vi "Autonomous Independent.vi"() -> ()   [LabVIEW 2016]
doc: "This VI is called when autonomous begins, and will automatically be terminated when autonomous ends. You can carry out timed or sensor driven robot movement independently without needing to return to the caller."
uses:
  <vilib>/Rock Robotics/WPI/ThirdParty/CanMotor/TalonSRX/WPI_CANTalonSRX_GlobalStatus.ctl
  <vilib>/Rock Robotics/WPI/SafetyOutput/WPI_SafetyOutputConfigMenu.ctl
panel:
  in  "y":dbl
  in  "Distance 2":dbl=6.462
  in  "Effort 2":dbl=0.5 format="%#_13g"
  out "Talon SRX Status 2":T1
  out "Talon SRX Status":T1
  in  "Effort 1":dbl=0.5 format="%#_13g"
  in  "Distance 1":dbl=6.462
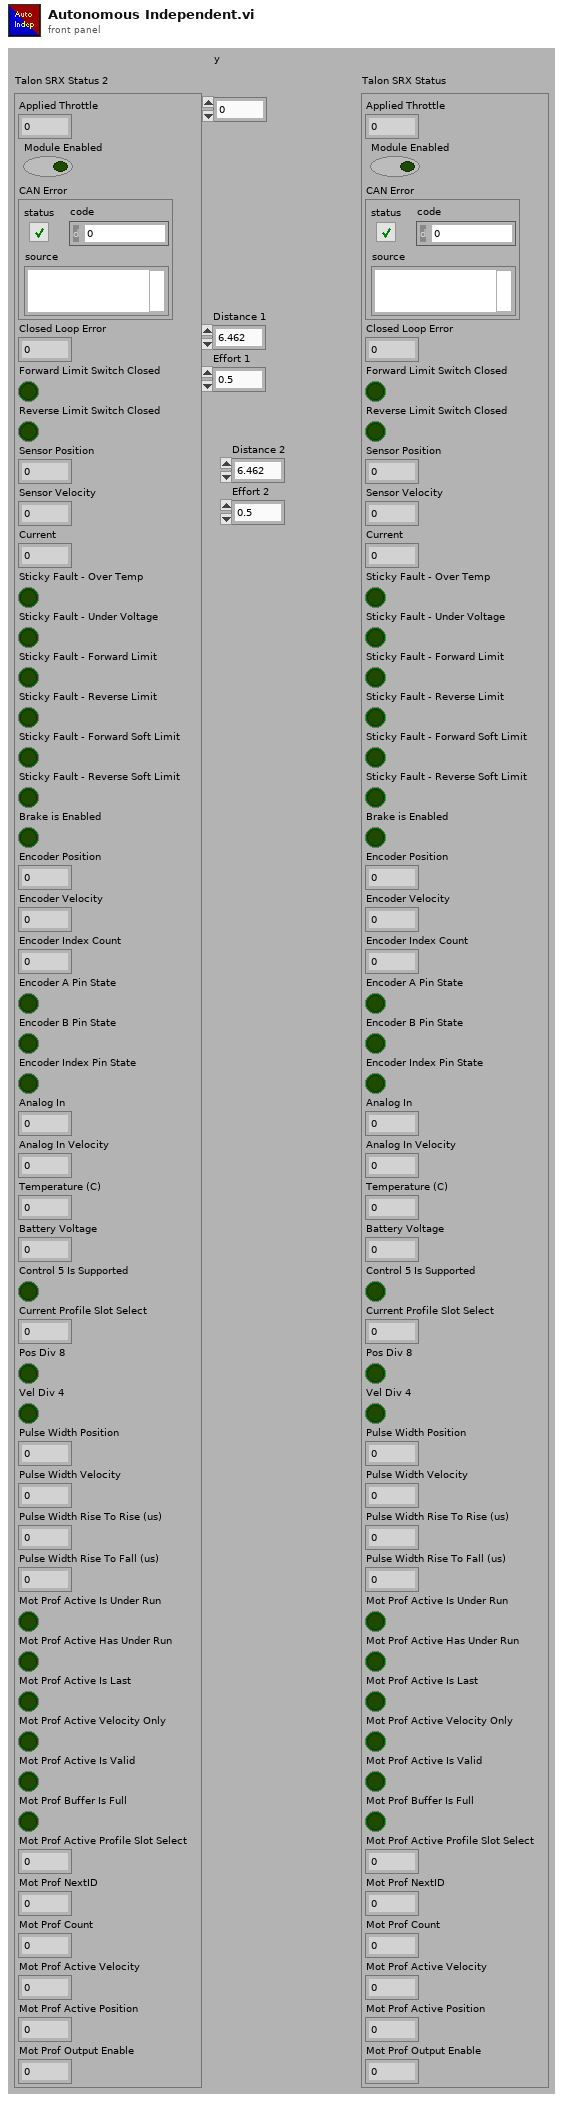
[diagram p1: front panel]
types:
  T1 = typedef "WPI_CANTalonSRX_GlobalStatus.ctl" = cluster{"Applied Throttle":dbl, "Module Enabled":bool, "CAN Error":errorcluster, "Closed Loop Error":dbl, "Forward Limit Switch Closed":bool, "Reverse Limit Switch Closed":bool, "Sensor Position":dbl, "Sensor Velocity":dbl, "Current":dbl, "Sticky Fault - Over Temp":bool, "Sticky Fault - Under Voltage":bool, "Sticky Fault - Forward Limit":bool, "Sticky Fault - Reverse Limit":bool, "Sticky Fault - Forward Soft Limit":bool, "Sticky Fault - Reverse Soft Limit":bool, "Brake is Enabled":bool, "Encoder Position":dbl, "Encoder Velocity":dbl, "Encoder Index Count":dbl, "Encoder A Pin State":bool, "Encoder B Pin State":bool, "Encoder Index Pin State":bool, "Analog In":dbl, "Analog In Velocity":dbl, "Temperature (C)":dbl, "Battery Voltage":dbl, "Control 5 Is Supported":bool, "Current Profile Slot Select":dbl, "Pos Div 8":bool, "Vel Div 4":bool, "Pulse Width Position":i32, "Pulse Width Velocity":i32, "Pulse Width Rise To Rise (us)":i32, "Pulse Width Rise To Fall (us)":i32, "Mot Prof Active Is Under Run":bool, "Mot Prof Active Has Under Run":bool, "Mot Prof Active Is Last":bool, "Mot Prof Active Velocity Only":bool, "Mot Prof Active Is Valid":bool, "Mot Prof Buffer Is Full":bool, "Mot Prof Active Profile Slot Select":i32, "Mot Prof NextID":i32, "Mot Prof Count":i32, "Mot Prof Active Velocity":dbl, "Mot Prof Active Position":dbl, "Mot Prof Output Enable":i32}
  T2 = typedef "WPI_SafetyOutputConfigMenu.ctl" = enum16{"Enable", "Disable"}
  T3 = typedef "WPI_MotorControlDeviceRef.ctl" = cluster{"DeviceStatus":errorcluster, "Type":T4, "PWM":cluster{"PWM Channel":T5, "DeadBand":T6}, "CAN":cluster{"Device Number":u8, "SetOutput VI Ref":variant, "GetOutput VI Ref":variant, "Enable VI Ref":variant, "Disable VI Ref":variant, "Data":variant}, "Invert":bool}
  T4 = typedef "WPI_MotorControlType.ctl" = enum16{"PWM", "CAN"}
  T5 = typedef "FPGA_DIOPWMChannel.ctl" = enum8{"PWM 0", "PWM 1", "PWM 2", "PWM 3", "PWM 4", "PWM 5", "PWM 6", "PWM 7", "PWM 8", "PWM 9", "PWM MXP 0", "PWM MXP 1", "PWM MXP 2", "PWM MXP 3", "PWM MXP 4", "PWM MXP 5", "PWM MXP 6", "PWM MXP 7", "PWM MXP 8", "PWM MXP 9", "Invalid"}
  T6 = typedef "WPI_PWMDeadband.ctl" = cluster{"Name":string, "maxPositivePwm":i32, "minPositivePwm":i32, "centerPwm":i32, "maxNegativePwm":i32, "minNegativePwm":i32, "angularRange":u16}
  T7 = typedef "WPI_GyroDevRef.ctl" = cluster{"DevStatus":errorcluster, "Analog Channel":T8, "Offset":dbl, "Gain (VoltsPerDegree/Second)":dbl, "Gyro Type":enum16{"Analog", "XRS450"}, "Handle":i32, "SPI Bus":T9, "Device Found":bool, "Sample Rate":dbl, "Calibrate On Open":bool}
  T8 = typedef "FPGA_AIChannel.ctl" = enum8{"AI 0", "AI 1", "AI 2", "AI 3", "AI MXP 0", "AI MXP 1", "AI MXP 2", "AI MXP 3", "Invalid"}
  T9 = typedef "spi_bus.ctl" = enum16{"SPI On-Board, CS0", "SPI On-Board, CS1", "SPI On-Board, CS2", "SPI On-Board, CS3", "SPI MXP", "Invalid"}
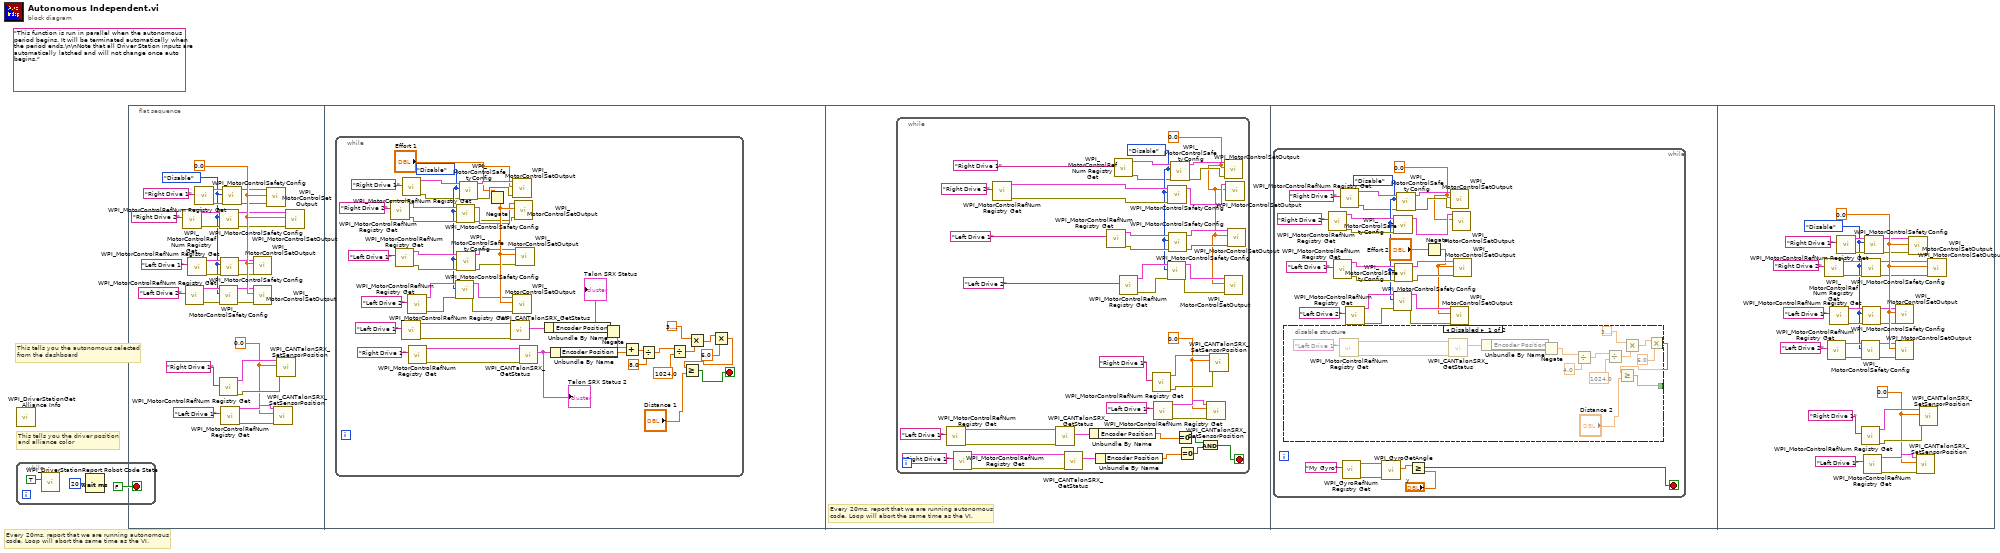
[diagram p0: block diagram]
diagram:
  (unwired) "This function is run in parallel when the autonomous period begins. It will be terminated automatically when the period ends.\n\nNote that all Driver Station inputs are automatically latched and will not change once auto begins."
  # "This tells you the autonomous selected\nfrom the dashboard"
  # "Every 20ms, report that we are running autonomous\ncode. Loop will abort the same time as the VI."
  # "This tells you the driver position\nand alliance color"
  n1 = while {
    stop <- FALSE stop-if-true
    n2 = call <vilib>:"WPI_DriverStationReport Robot Code State.vi"("Autonomous"=TRUE) -> ()  [unwired: 10 in, 1 out]
    n3 = Wait (ms)(milliseconds to wait=u32 20) -> ()  [unwired: 1 out]
  }
  n4 = call <vilib>:"WPI_DriverStationGet Alliance Info.vi"() -> ()  [unwired: 12 out]
  n5 = flat-sequence {
    frame #0 {
      w12 = WPI_SafetyOutputConfigMenu."Disable" ("mode")
      w21 = 0.0 ("Effort 2")
      w26 = 0.0 ("New Sensor Position")
      n6 = call <vilib>:"WPI_MotorControlRefNum Registry Get.vi"("refnum name"="Right Drive 2") -> ("error out"=w17:errorcluster, "MotorControlDevRef"=w18:T3)  [unwired: 9 in]
      n7 = call <vilib>:"WPI_MotorControlRefNum Registry Get.vi"("refnum name"="Left Drive 2") -> ("error out"=w13:errorcluster, "MotorControlDevRef"=w14:T3)  [unwired: 9 in]
      n8 = call <vilib>:"WPI_MotorControlRefNum Registry Get.vi"("refnum name"="Left Drive 1") -> ("error out"=w15:errorcluster, "MotorControlDevRef"=w16:T3)  [unwired: 9 in]
      n9 = call <vilib>:"WPI_MotorControlRefNum Registry Get.vi"("refnum name"="Right Drive 1") -> ("error out"=w20:errorcluster, "MotorControlDevRef"=w19:T3)  [unwired: 9 in]
      n10 = call <vilib>:"WPI_MotorControlSafetyConfig.vi"("error in (no error)"=w13, "mode"=w12, "MotorControlDevRef"=w14) -> ("error out"=w4:errorcluster, "MotorControlDevRef"=w5:T3)  [unwired: 7 in]
      n11 = call <vilib>:"WPI_MotorControlRefNum Registry Get.vi"("refnum name"="Right Drive 1") -> ("error out"=w27:errorcluster, "MotorControlDevRef"=w28:T3)  [unwired: 9 in]
      n12 = call <vilib>:"WPI_MotorControlSafetyConfig.vi"("error in (no error)"=w17, "mode"=w12, "MotorControlDevRef"=w18) -> ("error out"=w8:errorcluster, "MotorControlDevRef"=w9:T3)  [unwired: 7 in]
      n13 = call <vilib>:"WPI_MotorControlSafetyConfig.vi"("error in (no error)"=w15, "mode"=w12, "MotorControlDevRef"=w16) -> ("error out"=w6:errorcluster, "MotorControlDevRef"=w7:T3)  [unwired: 7 in]
      n14 = call <vilib>:"WPI_MotorControlRefNum Registry Get.vi"("refnum name"="Left Drive 1") -> ("error out"=w29:errorcluster, "MotorControlDevRef"=w30:T3)  [unwired: 9 in]
      n15 = call <vilib>:"WPI_MotorControlSafetyConfig.vi"("error in (no error)"=w20, "mode"=w12, "MotorControlDevRef"=w19) -> ("error out"=w10:errorcluster, "MotorControlDevRef"=w11:T3)  [unwired: 7 in]
      n16 = call <vilib>:"WPI_MotorControlSetOutput.vi"("error in (no error)"=w6, "Output"=w21, "MotorControlDevRef"=w7) -> ()  [unwired: 6 in, 3 out]
      n17 = call <vilib>:"WPI_MotorControlSetOutput.vi"("error in (no error)"=w4, "Output"=w21, "MotorControlDevRef"=w5) -> ()  [unwired: 6 in, 3 out]
      n18 = call <vilib>:"WPI_MotorControlSetOutput.vi"("error in (no error)"=w10, "Output"=w21, "MotorControlDevRef"=w11) -> ()  [unwired: 6 in, 3 out]
      n19 = call <vilib>:"WPI_CANTalonSRX_SetSensorPosition.vi"("error in (no error)"=w29, "New Sensor Position"=w26, "CAN Talon SRX Ref"=w30) -> ()  [unwired: 7 in, 2 out]
      n20 = call <vilib>:"WPI_CANTalonSRX_SetSensorPosition.vi"("error in (no error)"=w27, "New Sensor Position"=w26, "CAN Talon SRX Ref"=w28) -> ()  [unwired: 7 in, 2 out]
      n21 = call <vilib>:"WPI_MotorControlSetOutput.vi"("error in (no error)"=w8, "Output"=w21, "MotorControlDevRef"=w9) -> ()  [unwired: 6 in, 3 out]
    }
    frame #1 {
      n22 = while {
        stop <- w42 stop-if-true
        w48 = WPI_SafetyOutputConfigMenu."Disable" ("mode")
        n23 = call <vilib>:"WPI_MotorControlRefNum Registry Get.vi"("refnum name"="Right Drive 2") -> ("error out"=w51:errorcluster, "MotorControlDevRef"=w52:T3)  [unwired: 9 in]
        n24 = call <vilib>:"WPI_MotorControlRefNum Registry Get.vi"("refnum name"="Left Drive 1") -> ("error out"=w55:errorcluster, "MotorControlDevRef"=w56:T3)  [unwired: 9 in]
        n25 = call <vilib>:"WPI_MotorControlRefNum Registry Get.vi"("refnum name"="Left Drive 1") -> ("error out"=w76:errorcluster, "MotorControlDevRef"=w77:T3)  [unwired: 9 in]
        n26 = call <vilib>:"WPI_MotorControlRefNum Registry Get.vi"("refnum name"="Right Drive 1") -> ("error out"=w46:errorcluster, "MotorControlDevRef"=w63:T3)  [unwired: 9 in]
        n27 = call <vilib>:"WPI_MotorControlRefNum Registry Get.vi"("refnum name"="Left Drive 2") -> ("error out"=w59:errorcluster, "MotorControlDevRef"=w60:T3)  [unwired: 9 in]
        n28 = call <vilib>:"WPI_MotorControlRefNum Registry Get.vi"("refnum name"="Right Drive 1") -> ("error out"=w40:errorcluster, "MotorControlDevRef"=w74:T3)  [unwired: 9 in]
        n29 = call <vilib>:"WPI_MotorControlSafetyConfig.vi"("error in (no error)"=w59, "mode"=w48, "MotorControlDevRef"=w60) -> ("error out"=w57:errorcluster, "MotorControlDevRef"=w58:T3)  [unwired: 7 in]
        n30 = call <vilib>:"WPI_MotorControlSafetyConfig.vi"("error in (no error)"=w51, "mode"=w48, "MotorControlDevRef"=w52) -> ("error out"=w49:errorcluster, "MotorControlDevRef"=w50:T3)  [unwired: 7 in]
        n31 = call <vilib>:"WPI_MotorControlSafetyConfig.vi"("error in (no error)"=w55, "mode"=w48, "MotorControlDevRef"=w56) -> ("error out"=w53:errorcluster, "MotorControlDevRef"=w54:T3)  [unwired: 7 in]
        n32 = call <vilib>:"WPI_MotorControlSafetyConfig.vi"("error in (no error)"=w46, "mode"=w48, "MotorControlDevRef"=w63) -> ("error out"=w47:errorcluster, "MotorControlDevRef"=w62:T3)  [unwired: 7 in]
        n33 = Negate(x="Effort 1") -> (-x=w61:dbl)
        n34 = call <vilib>:"WPI_CANTalonSRX_GetStatus.vi"("error in (no error)"=w76, "CAN Talon SRX Ref"=w77) -> ("Talon SRX Status"=w75:T1)  [unwired: 7 in, 2 out]
        "Talon SRX Status" <- w75
        n35 = call <vilib>:"WPI_MotorControlSetOutput.vi"("error in (no error)"=w47, "Output"="Effort 1", "MotorControlDevRef"=w62) -> ()  [unwired: 6 in, 3 out]
        n36 = call <vilib>:"WPI_MotorControlSetOutput.vi"("error in (no error)"=w57, "Output"=w61, "MotorControlDevRef"=w58) -> ()  [unwired: 6 in, 3 out]
        n37 = call <vilib>:"WPI_MotorControlSetOutput.vi"("error in (no error)"=w49, "Output"=w61, "MotorControlDevRef"=w50) -> ()  [unwired: 6 in, 3 out]
        n38 = call <vilib>:"WPI_MotorControlSetOutput.vi"("error in (no error)"=w53, "Output"=w61, "MotorControlDevRef"=w54) -> ()  [unwired: 6 in, 3 out]
        n39 = call <vilib>:"WPI_CANTalonSRX_GetStatus.vi"("error in (no error)"=w40, "CAN Talon SRX Ref"=w74) -> ("Talon SRX Status"=w44:T1)  [unwired: 7 in, 2 out]
        "Talon SRX Status 2" <- w44
        n40 = Unbundle By Name(w75) -> ("Encoder Position"=w66:dbl)
        n41 = Unbundle By Name(w44) -> ("Encoder Position"=w67:dbl)
        n42 = Negate(x=w66) -> (-x=w43:dbl)
        n43 = Add(x=w43, y=w67) -> (x+y=w65:dbl)
        n44 = Divide(x=w65, y=8.0) -> (x/y=w39:dbl)
        n45 = Divide(x=w39, y=1024.0) -> (x/y=w36:dbl)
        n46 = Multiply(x=3.141592653589793, y=w36) -> (x*y=w37:dbl)
        n47 = Multiply(x=w37, y=6.0) -> (x*y=w33:dbl)
        n48 = Greater Or Equal?(x=w33, y="Distance 1") -> (x >= y?=w42:bool)
      }
    }
    frame #2 {
      # "Every 20ms, report that we are running autonomous\ncode. Loop will abort the same time as the VI."
      n49 = while {
        stop <- w78 stop-if-true
        w91 = 0.0
        w95 = WPI_SafetyOutputConfigMenu."Disable" ("mode")
        w112 = 0.0 ("New Sensor Position")
        n50 = call <vilib>:"WPI_MotorControlRefNum Registry Get.vi"("refnum name"="Left Drive 1") -> ("error out"=w89:errorcluster, "MotorControlDevRef"=w90:T3)  [unwired: 9 in]
        n51 = call <vilib>:"WPI_MotorControlRefNum Registry Get.vi"("refnum name"="Right Drive 1") -> ("error out"=w83:errorcluster, "MotorControlDevRef"=w87:T3)  [unwired: 9 in]
        n52 = call <vilib>:"WPI_MotorControlRefNum Registry Get.vi"("refnum name"="Right Drive 2") -> ("error out"=w96:errorcluster, "MotorControlDevRef"=w97:T3)  [unwired: 9 in]
        n53 = call <vilib>:"WPI_CANTalonSRX_GetStatus.vi"("error in (no error)"=w89, "CAN Talon SRX Ref"=w90) -> ("Talon SRX Status"=w88:T1)  [unwired: 7 in, 2 out]
        n54 = call <vilib>:"WPI_CANTalonSRX_GetStatus.vi"("error in (no error)"=w83, "CAN Talon SRX Ref"=w87) -> ("Talon SRX Status"=w84:T1)  [unwired: 7 in, 2 out]
        n55 = Unbundle By Name(w88) -> ("Encoder Position"=w82:dbl)
        n56 = Unbundle By Name(w84) -> ("Encoder Position"=w80:dbl)
        n57 = call <vilib>:"WPI_MotorControlRefNum Registry Get.vi"("refnum name"="Left Drive 1") -> ("error out"=w100:errorcluster, "MotorControlDevRef"=w101:T3)  [unwired: 9 in]
        n58 = call <vilib>:"WPI_MotorControlRefNum Registry Get.vi"("refnum name"="Right Drive 1") -> ("error out"=w93:errorcluster, "MotorControlDevRef"=w107:T3)  [unwired: 9 in]
        n59 = call <vilib>:"WPI_MotorControlRefNum Registry Get.vi"("refnum name"="Left Drive 2") -> ("error out"=w104:errorcluster, "MotorControlDevRef"=w105:T3)  [unwired: 9 in]
        n60 = call <vilib>:"WPI_MotorControlRefNum Registry Get.vi"("refnum name"="Right Drive 1") -> ("error out"=w113:errorcluster, "MotorControlDevRef"=w114:T3)  [unwired: 9 in]
        n61 = call <vilib>:"WPI_MotorControlRefNum Registry Get.vi"("refnum name"="Left Drive 1") -> ("error out"=w115:errorcluster, "MotorControlDevRef"=w116:T3)  [unwired: 9 in]
        n62 = call <vilib>:"WPI_MotorControlSafetyConfig.vi"("error in (no error)"=w104, "mode"=w95, "MotorControlDevRef"=w105) -> ("error out"=w102:errorcluster, "MotorControlDevRef"=w103:T3)  [unwired: 7 in]
        n63 = call <vilib>:"WPI_MotorControlSafetyConfig.vi"("error in (no error)"=w96, "mode"=w95, "MotorControlDevRef"=w97) -> ("MotorControlDevRef"=w92:T3)  [unwired: 7 in, 1 out]
        n64 = call <vilib>:"WPI_MotorControlSafetyConfig.vi"("error in (no error)"=w100, "mode"=w95, "MotorControlDevRef"=w101) -> ("error out"=w98:errorcluster, "MotorControlDevRef"=w99:T3)  [unwired: 7 in]
        n65 = call <vilib>:"WPI_MotorControlSafetyConfig.vi"("error in (no error)"=w93, "mode"=w95, "MotorControlDevRef"=w107) -> ("error out"=w94:errorcluster, "MotorControlDevRef"=w106:T3)  [unwired: 7 in]
        n66 = Equal To 0?(x=w82) -> (x = 0?=w81:bool)
        n67 = Equal To 0?(x=w80) -> (x = 0?=w79:bool)
        n68 = And(x=w81, y=w79) -> (x .and. y?=w78:bool)
        n69 = call <vilib>:"WPI_CANTalonSRX_SetSensorPosition.vi"("error in (no error)"=w115, "New Sensor Position"=w112, "CAN Talon SRX Ref"=w116) -> ()  [unwired: 7 in, 2 out]
        n70 = call <vilib>:"WPI_CANTalonSRX_SetSensorPosition.vi"("error in (no error)"=w113, "New Sensor Position"=w112, "CAN Talon SRX Ref"=w114) -> ()  [unwired: 7 in, 2 out]
        n71 = call <vilib>:"WPI_MotorControlSetOutput.vi"("error in (no error)"=w94, "Output"=w91, "MotorControlDevRef"=w106) -> ()  [unwired: 6 in, 3 out]
        n72 = call <vilib>:"WPI_MotorControlSetOutput.vi"("error in (no error)"=w102, "Output"=w91, "MotorControlDevRef"=w103) -> ()  [unwired: 6 in, 3 out]
        n73 = call <vilib>:"WPI_MotorControlSetOutput.vi"("Output"=w91, "MotorControlDevRef"=w92) -> ()  [unwired: 7 in, 3 out]
        n74 = call <vilib>:"WPI_MotorControlSetOutput.vi"("error in (no error)"=w98, "Output"=w91, "MotorControlDevRef"=w99) -> ()  [unwired: 6 in, 3 out]
      }
    }
    frame #3 {
      n75 = while {
        stop <- w119 stop-if-true
        w127 = 0.0
        w131 = WPI_SafetyOutputConfigMenu."Disable" ("mode")
        n76 = disable-structure shown="Disabled" {
          disable-tunnel: [w157 _] -> _
          frame Disabled {
            n77 = call <vilib>:"WPI_MotorControlRefNum Registry Get.vi"("refnum name"="Left Drive 1") -> ("error out"=w162:errorcluster, "MotorControlDevRef"=w163:T3)  [unwired: 9 in]
            n78 = call <vilib>:"WPI_CANTalonSRX_GetStatus.vi"("error in (no error)"=w162, "CAN Talon SRX Ref"=w163) -> ("Talon SRX Status"=w161:T1)  [unwired: 7 in, 2 out]
            n79 = Unbundle By Name(w161) -> ("Encoder Position"=w159:dbl)
            n80 = Negate(x=w159) -> (-x=w149:dbl)
            n81 = Divide(x=w149, y=4.0) -> (x/y=w155:dbl)
            n82 = Divide(x=w155, y=1024.0) -> (x/y=w153:dbl)
            n83 = Multiply(x=3.141592653589793, y=w153) -> (x*y=w154:dbl)
            n84 = Multiply(x=w154, y=6.0) -> (x*y=w150:dbl)
            n85 = Greater Or Equal?(x=w150, y="Distance 2") -> (x >= y?=w157:bool)
          }
          frame Enabled {
          }
        }
        n86 = call <vilib>:"WPI_MotorControlRefNum Registry Get.vi"("refnum name"="Right Drive 2") -> ("error out"=w132:errorcluster, "MotorControlDevRef"=w133:T3)  [unwired: 9 in]
        n87 = call <vilib>:"WPI_MotorControlRefNum Registry Get.vi"("refnum name"="Left Drive 1") -> ("error out"=w136:errorcluster, "MotorControlDevRef"=w137:T3)  [unwired: 9 in]
        n88 = call <vilib>:"WPI_MotorControlRefNum Registry Get.vi"("refnum name"="Right Drive 1") -> ("error out"=w129:errorcluster, "MotorControlDevRef"=w143:T3)  [unwired: 9 in]
        n89 = call <vilib>:"WPI_GyroRefNum Registry Get.vi"("refnum name"="My Gyro") -> ("error out"=w124:errorcluster, "GyroDevRef"=w123:T7)  [unwired: 9 in]
        n90 = call <vilib>:"WPI_MotorControlRefNum Registry Get.vi"("refnum name"="Left Drive 2") -> ("error out"=w140:errorcluster, "MotorControlDevRef"=w141:T3)  [unwired: 9 in]
        n91 = call <vilib>:"WPI_GyroGetAngle.vi"("error in"=w124, "GyroDevRef"=w123) -> ("Angle"=w121:dbl)  [unwired: 5 in, 4 out]
        n92 = call <vilib>:"WPI_MotorControlSafetyConfig.vi"("error in (no error)"=w140, "mode"=w131, "MotorControlDevRef"=w141) -> ("error out"=w138:errorcluster, "MotorControlDevRef"=w139:T3)  [unwired: 7 in]
        n93 = call <vilib>:"WPI_MotorControlSafetyConfig.vi"("error in (no error)"=w132, "mode"=w131, "MotorControlDevRef"=w133) -> ("MotorControlDevRef"=w128:T3)  [unwired: 7 in, 1 out]
        n94 = call <vilib>:"WPI_MotorControlSafetyConfig.vi"("error in (no error)"=w136, "mode"=w131, "MotorControlDevRef"=w137) -> ("error out"=w134:errorcluster, "MotorControlDevRef"=w135:T3)  [unwired: 7 in]
        n95 = call <vilib>:"WPI_MotorControlSafetyConfig.vi"("error in (no error)"=w129, "mode"=w131, "MotorControlDevRef"=w143) -> ("error out"=w130:errorcluster, "MotorControlDevRef"=w142:T3)  [unwired: 7 in]
        n96 = Greater Or Equal?(x=w121, y="y") -> (x >= y?=w119:bool)
        n97 = Negate(x="Effort 2") -> (-x=w125:dbl)
        n98 = call <vilib>:"WPI_MotorControlSetOutput.vi"("error in (no error)"=w130, "Output"=w127, "MotorControlDevRef"=w142) -> ()  [unwired: 6 in, 3 out]
        n99 = call <vilib>:"WPI_MotorControlSetOutput.vi"("error in (no error)"=w138, "Output"=w125, "MotorControlDevRef"=w139) -> ()  [unwired: 6 in, 3 out]
        n100 = call <vilib>:"WPI_MotorControlSetOutput.vi"("Output"=w127, "MotorControlDevRef"=w128) -> ()  [unwired: 7 in, 3 out]
        n101 = call <vilib>:"WPI_MotorControlSetOutput.vi"("error in (no error)"=w134, "Output"=w125, "MotorControlDevRef"=w135) -> ()  [unwired: 6 in, 3 out]
      }
    }
    frame #4 {
      w172 = WPI_SafetyOutputConfigMenu."Disable" ("mode")
      w181 = 0.0 ("Effort 2")
      w186 = 0.0 ("New Sensor Position")
      n102 = call <vilib>:"WPI_MotorControlRefNum Registry Get.vi"("refnum name"="Right Drive 2") -> ("error out"=w177:errorcluster, "MotorControlDevRef"=w178:T3)  [unwired: 9 in]
      n103 = call <vilib>:"WPI_MotorControlRefNum Registry Get.vi"("refnum name"="Left Drive 2") -> ("error out"=w173:errorcluster, "MotorControlDevRef"=w174:T3)  [unwired: 9 in]
      n104 = call <vilib>:"WPI_MotorControlRefNum Registry Get.vi"("refnum name"="Left Drive 1") -> ("error out"=w175:errorcluster, "MotorControlDevRef"=w176:T3)  [unwired: 9 in]
      n105 = call <vilib>:"WPI_MotorControlRefNum Registry Get.vi"("refnum name"="Right Drive 1") -> ("error out"=w180:errorcluster, "MotorControlDevRef"=w179:T3)  [unwired: 9 in]
      n106 = call <vilib>:"WPI_MotorControlSafetyConfig.vi"("error in (no error)"=w173, "mode"=w172, "MotorControlDevRef"=w174) -> ("error out"=w164:errorcluster, "MotorControlDevRef"=w165:T3)  [unwired: 7 in]
      n107 = call <vilib>:"WPI_MotorControlRefNum Registry Get.vi"("refnum name"="Right Drive 1") -> ("error out"=w187:errorcluster, "MotorControlDevRef"=w188:T3)  [unwired: 9 in]
      n108 = call <vilib>:"WPI_MotorControlSafetyConfig.vi"("error in (no error)"=w177, "mode"=w172, "MotorControlDevRef"=w178) -> ("error out"=w168:errorcluster, "MotorControlDevRef"=w169:T3)  [unwired: 7 in]
      n109 = call <vilib>:"WPI_MotorControlSafetyConfig.vi"("error in (no error)"=w175, "mode"=w172, "MotorControlDevRef"=w176) -> ("error out"=w166:errorcluster, "MotorControlDevRef"=w167:T3)  [unwired: 7 in]
      n110 = call <vilib>:"WPI_MotorControlRefNum Registry Get.vi"("refnum name"="Left Drive 1") -> ("error out"=w189:errorcluster, "MotorControlDevRef"=w190:T3)  [unwired: 9 in]
      n111 = call <vilib>:"WPI_MotorControlSafetyConfig.vi"("error in (no error)"=w180, "mode"=w172, "MotorControlDevRef"=w179) -> ("error out"=w170:errorcluster, "MotorControlDevRef"=w171:T3)  [unwired: 7 in]
      n112 = call <vilib>:"WPI_MotorControlSetOutput.vi"("error in (no error)"=w166, "Output"=w181, "MotorControlDevRef"=w167) -> ()  [unwired: 6 in, 3 out]
      n113 = call <vilib>:"WPI_MotorControlSetOutput.vi"("error in (no error)"=w164, "Output"=w181, "MotorControlDevRef"=w165) -> ()  [unwired: 6 in, 3 out]
      n114 = call <vilib>:"WPI_MotorControlSetOutput.vi"("error in (no error)"=w170, "Output"=w181, "MotorControlDevRef"=w171) -> ()  [unwired: 6 in, 3 out]
      n115 = call <vilib>:"WPI_CANTalonSRX_SetSensorPosition.vi"("error in (no error)"=w189, "New Sensor Position"=w186, "CAN Talon SRX Ref"=w190) -> ()  [unwired: 7 in, 2 out]
      n116 = call <vilib>:"WPI_CANTalonSRX_SetSensorPosition.vi"("error in (no error)"=w187, "New Sensor Position"=w186, "CAN Talon SRX Ref"=w188) -> ()  [unwired: 7 in, 2 out]
      n117 = call <vilib>:"WPI_MotorControlSetOutput.vi"("error in (no error)"=w168, "Output"=w181, "MotorControlDevRef"=w169) -> ()  [unwired: 6 in, 3 out]
    }
  }
